vi "NI-Embedded CAN for RIO subVI - CAN Frame to Table test.vi"(5 "Boolean":bool, 7 "Hexadecimal?":bool, 8 "x":dbl, 9 "timestamp":timestamp, 10 "Input Array":string[][](array[string]), 11 "CAN frame":T1 {"type" items=["CAN Data", "CAN Remote"]; "identifier" format="%.0x"}) -> (0 "Numeric":dbl, 1 "(hi.lo)":u16(knob) scale=0.0..4095.0, 2 "string":string, 3 "Output Array":string[][](array[string]), 6 "okres 100":dbl)   [LabVIEW 2014]
doc: "This example shows how to put a CAN transceiver to sleep on RIO Embedded CAN devices."
uses:
  K/CANFrameControl.ctl
panel:
  out "subarray 2":string[](array[string])
  out "subarray":string[](array[string])
  in  "Array":T1[](array[typedef]) {"type" items=["CAN Data", "CAN Remote"]; "identifier" format="%.0x"}
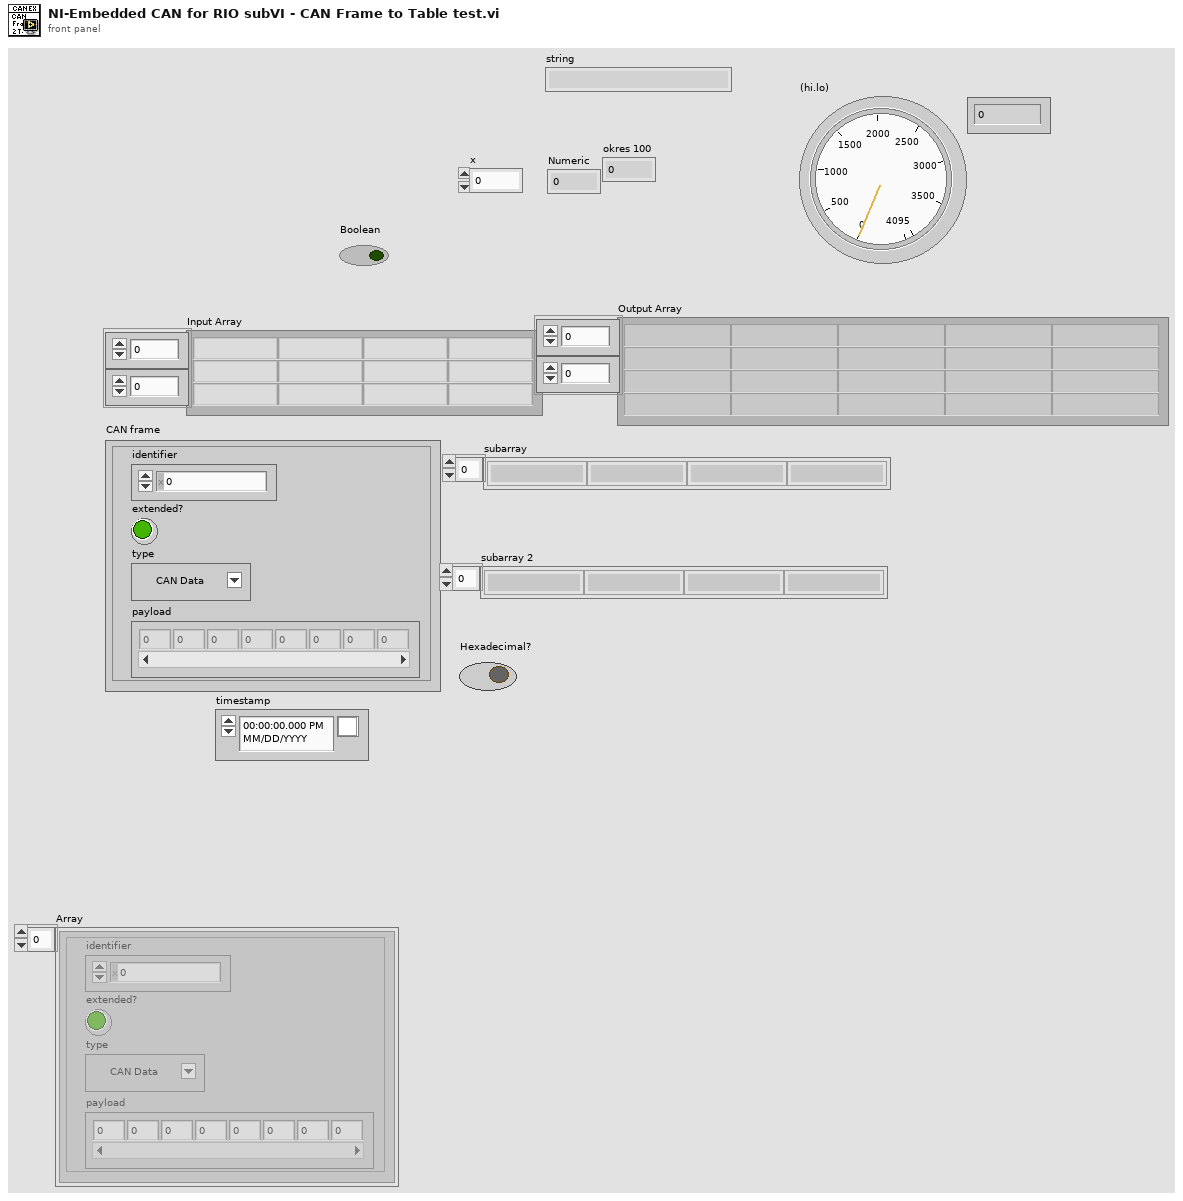
[diagram p1: front panel]
types:
  T1 = typedef "CANFrameControl.ctl" = cluster{"identifier":u32, "extended?":bool, "type":u8, "payload":u8[]}
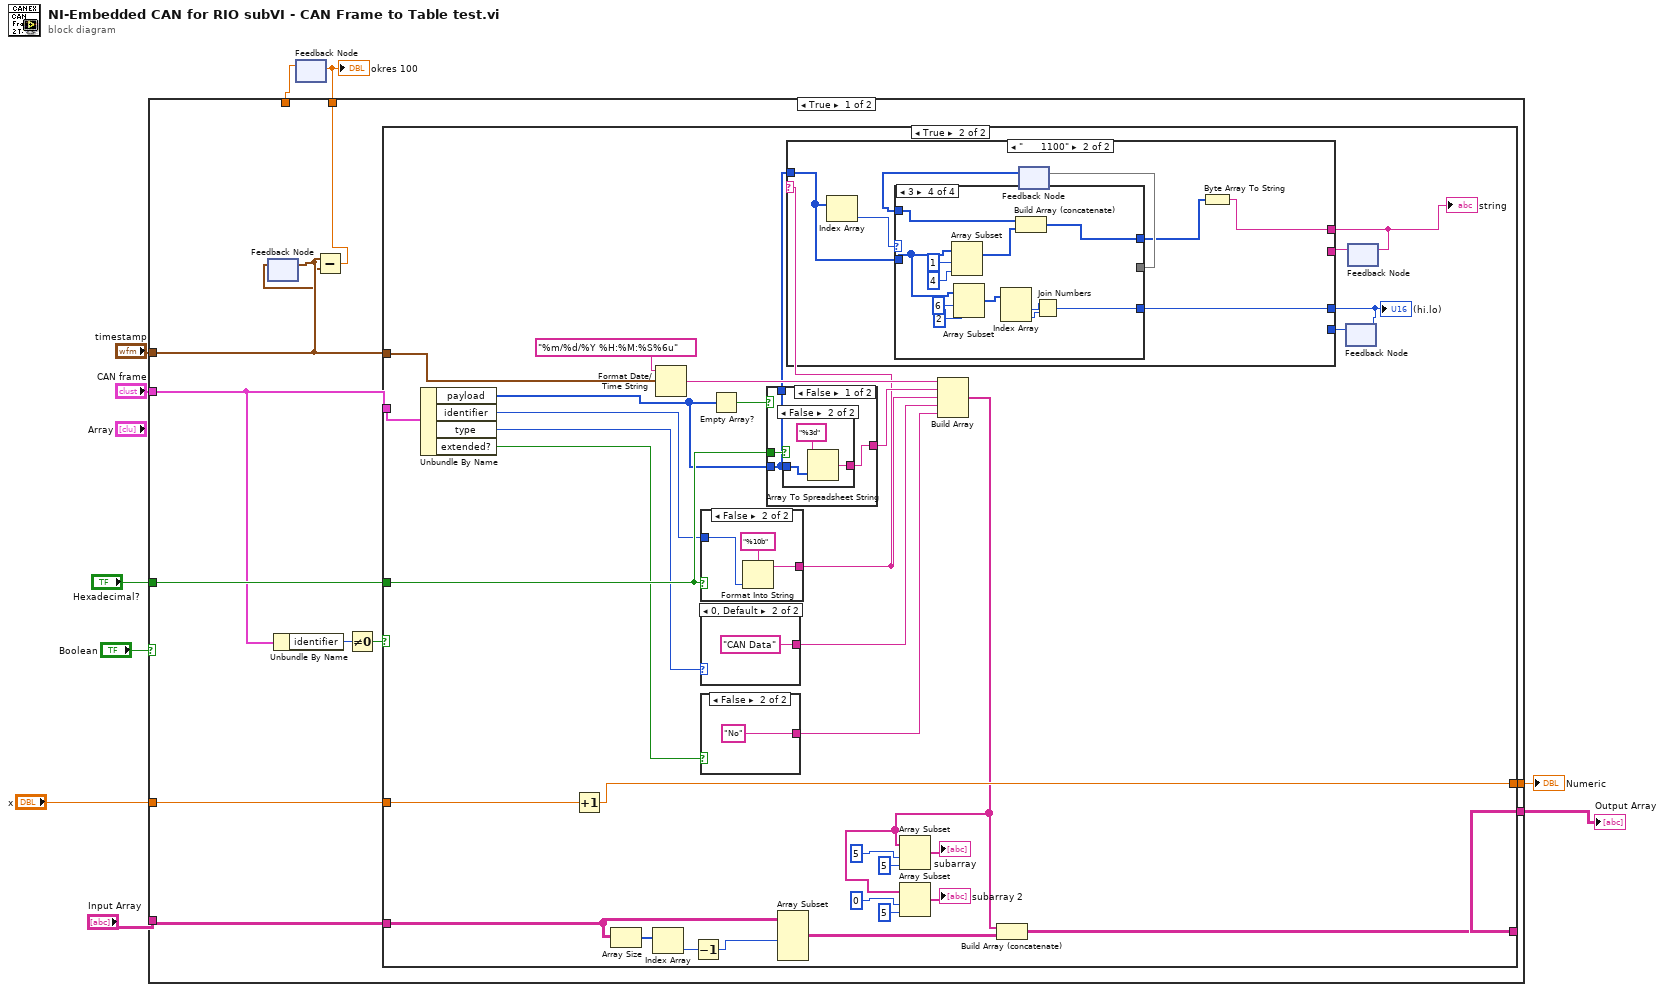
[diagram p0: block diagram]
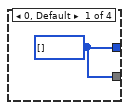
[diagram p4: hidden frame]
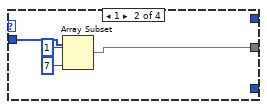
[diagram p5: hidden frame]
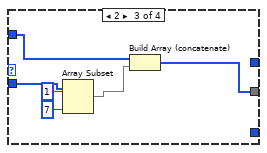
[diagram p6: hidden frame]
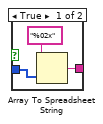
[diagram p7: hidden frame]
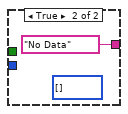
[diagram p8: hidden frame]
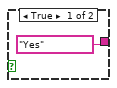
[diagram p9: hidden frame]
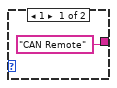
[diagram p10: hidden frame]
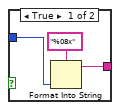
[diagram p11: hidden frame]
diagram:
  n1 = feedback #1() -> (w1:dbl)  [unwired: 1 in]
  n2 = case shown="True" "Boolean" {
    tunnel: "Input Array" -> [w19 w112]
    tunnel: [w21 w112] -> w7
    tunnel: "Hexadecimal?" -> [w20 _]
    tunnel: "CAN frame" -> [w16 _]
    tunnel: "timestamp" -> [w12 _]
    tunnel: [w18 w111] -> w4
    tunnel: "x" -> [w17 w111]
    tunnel: [w13 w110] -> w2
    tunnel: w1 -> [_ w110]
    frame True {
      n3 = feedback #2() -> (w11:timestamp)  [unwired: 1 in]
      n4 = feedback-in #2(w12) -> ()
      n5 = Unbundle By Name(w16) -> ("identifier"=w15:u32)
      n6 = Subtract(x=w12, y=w11) -> (x-y=w13:dbl)
      n7 = Not Equal To 0?(x=w15) -> (x != 0?=w14:bool)
      n8 = case shown="True" w14 {
        tunnel: [w22 w57] -> w21
        tunnel: w20 -> [_ w56]
        tunnel: w12 -> [_ w31]
        tunnel: w19 -> [w22 w55]
        tunnel: w16 -> [_ w54]
        tunnel: [w23 w53] -> w18
        tunnel: w17 -> [w23 w52]
        frame False {
        }
        frame True {
          n9 = Unbundle By Name(w54) -> ("payload"=w30:u8[], "identifier"=w32:u32, "type"=w41:u8, "extended?"=w38:bool)
          n10 = Increment(x=w52) -> (x+1=w53:dbl)
          n11 = Array Size(array=w55) -> (size(s)=w51:i32[])
          n12 = Index Array(array=w51) -> (element=w50:i32)  [unwired: 1 in]
          n13 = Format Date/Time String(time format string (%c)="%m/%d/%Y %H:%M:%S%6u", seconds (now)=w31) -> (date/time string=w42:string)  [unwired: 1 in]
          n14 = Decrement(x=w50) -> (x-1=w33:i32)
          n15 = case shown="False" w56 {
            tunnel: w32 -> [w105 w108]
            tunnel: [w104 w107] -> w29
            frame True {
              n16 = Format Into String(format string="%08x", w105) -> (resulting string=w104:string)  [unwired: 2 in, 1 out]
            }
            frame False {
              n17 = Format Into String(format string="%10b", w108) -> (resulting string=w107:string)  [unwired: 2 in, 1 out]
            }
          }
          n18 = case shown="0, Default" w41 {
            tunnel: ["CAN Remote" "CAN Data"] -> w40
            frame 1 {
            }
            frame 0, Default {
            }
          }
          n19 = case shown="False" w38 {
            tunnel: ["Yes" "No"] -> w39
            frame True {
            }
            frame False {
            }
          }
          n20 = Empty Array?(array=w30) -> (empty?=w35:bool)
          n21 = case shown="False" w35 {
            tunnel: [w91 "No Data"] -> w37
            tunnel: w30 -> [w90 _]
            tunnel: w56 -> [w92 _]
            tunnel: [w90 _] -> w28
            frame False {
              n22 = case shown="False" w92 {
                tunnel: w90 -> [w93 w96]
                tunnel: [w94 w97] -> w91
                frame True {
                  n23 = Array To Spreadsheet String(array=w93, 3:"%02x" ("format string")) -> (spreadsheet string=w94:string)  [unwired: 1 in]
                }
                frame False {
                  n24 = Array To Spreadsheet String(array=w96, 3:"%3d" ("format string")) -> (spreadsheet string=w97:string)  [unwired: 1 in]
                }
              }
            }
            frame True {
              (unwired) u8[] [] ("payload")
            }
          }
          n25 = Array Subset(array=w55, length (row)=w33) -> (w43:string[][])  [unwired: 3 in]
          n26 = Build Array(w42, w37, w29, w40, w39) -> (w34:string[])
          n27 = Array Subset(array=w34, index=5 ("length"), length=5) -> (→"subarray":string[])
          n28 = Array Subset(array=w34, index=0 ("length"), length=5) -> (→"subarray 2":string[])
          n29 = Build Array (concatenate)(w34, w43) -> (w57:string[][])
          n30 = feedback #3() -> (w24:u16)  [unwired: 1 in]
          n31 = feedback #4() -> (w26:string)  [unwired: 1 in]
          n32 = case shown="\"      1100\"" w29 {
            tunnel: w28 -> [_ w65]
            tunnel: [w59 w61] -> w27
            tunnel: w26 -> [w59 _]
            tunnel: [w58 w60] -> w25
            tunnel: w24 -> [w58 _]
            frame "False", Default {
            }
            frame "      1100" {
              n33 = Index Array(array=w65) -> (element=w66:u8)  [unwired: 1 in]
              n34 = feedback #5() -> (w63:u8[])  [unwired: 1 in]
              n35 = case shown="3" w66 {
                tunnel: w65 -> [_ w69 w75 w84]
                tunnel: [w67 w68 w72 _] -> w64
                tunnel: w63 -> [_ _ w74 w88]
                tunnel: [w67 _ _ w87] -> w62
                tunnel: [_ _ _ w78] -> w60
                frame 0, Default {
                  w67 = u8[] []
                }
                frame 1 {
                  n36 = Array Subset(array=w69, index=1, length=7) -> (w68:u8[])
                }
                frame 2 {
                  n37 = Array Subset(array=w75, index=1, length=7) -> (w73:u8[])
                  n38 = Build Array (concatenate)(w74, w73) -> (w72:u8[])
                }
                frame 3 {
                  n39 = Array Subset(array=w84, index=1, length=4) -> (w86:u8[])
                  n40 = Array Subset(array=w84, index=6, length=2) -> (w81:u8[])
                  n41 = Index Array(array=w81) -> (element #1=w80:u8, element #2=w79:u8)  [unwired: 2 in]
                  n42 = Build Array (concatenate)(w88, w86) -> (w87:u8[])
                  n43 = Join Numbers(hi=w80, lo=w79) -> ((hi.lo)=w78:u16)
                }
              }
              n44 = feedback-in #5(w64) -> ()
              n45 = Byte Array To String(unsigned byte array=w62) -> (string=w61:string)
            }
          }
          "string" <- w27
          "(hi.lo)" <- w25
          n46 = feedback-in #3(w25) -> ()
          n47 = feedback-in #4(w27) -> ()
        }
      }
    }
    frame False {
    }
  }
  "Output Array" <- w7
  "Numeric" <- w4
  "okres 100" <- w2
  n48 = feedback-in #1(w2) -> ()
